vi "helper.vi"(8 "error in (no error)":errorcluster) -> (0 "error out":errorcluster, 2 "Application:All VIs In Memory":string[](array[string]))   [LabVIEW 2016]
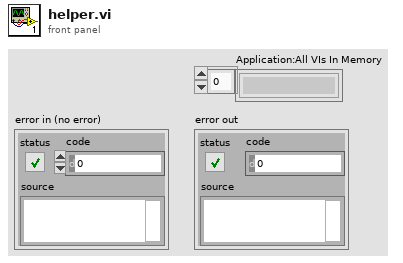
[diagram p1: front panel]
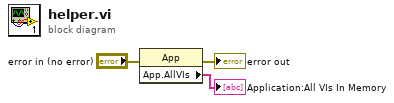
[diagram p0: block diagram]
diagram:
  n1 = property class="App"(error in="error in (no error)") -> (error out=→"error out":errorcluster, "App.AllVIs"=→"Application:All VIs In Memory":string[])  [unwired: 1 in, 1 out]
